vi "Read connections.vi"(8 "error in (no error)":errorcluster, 11 "Baseline Mocon piD-Tech plus in":refnum<class "Baseline Mocon piD-Tech plus.lvclass">) -> (0 "error out":errorcluster, 2 "Baseline-Mocon piD-TECH plus":T1, 3 "Baseline Mocon piD-Tech plus out":refnum<class "Baseline Mocon piD-Tech plus.lvclass">)   [LabVIEW 2011, in "Baseline Mocon piD-Tech plus.lvclass"]
uses:
  Baseline Mocon piD-Tech plus.lvclass
  Connections.ctl
  Baseline Mocon piD-Tech plus.lvclass/Baseline Mocon piD-Tech plus.ctl
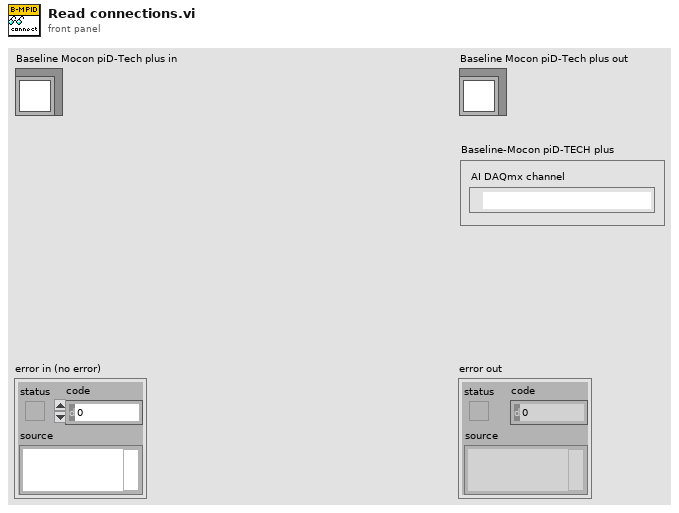
[diagram p1: front panel]
types:
  T1 = typedef "Baseline Mocon piD-Tech plus.lvclass/Connections.ctl" = cluster{"AI DAQmx channel":tag}
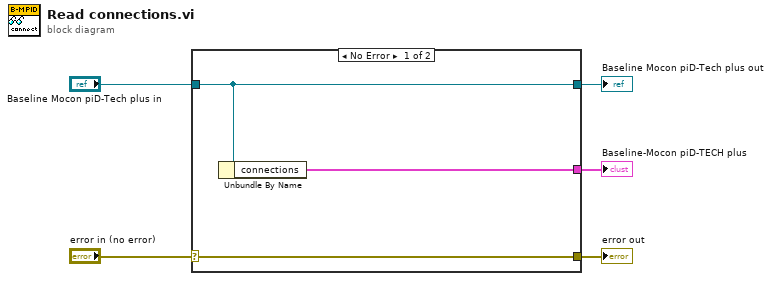
[diagram p0: block diagram]
diagram:
  n1 = case shown="No Error" "error in (no error)" {
    selector: "error in (no error)" -> [w8 w9]
    tunnel: [w8 w9] -> w4
    tunnel: [w7 w10] -> w2
    tunnel: "Baseline Mocon piD-Tech plus in" -> [w7 w10]
    tunnel: [w6 _] -> w1
    frame No Error {
      n2 = Unbundle By Name(w7) -> ("connections"=w6:T1)
    }
    frame Error {
    }
  }
  "error out" <- w4
  "Baseline Mocon piD-Tech plus out" <- w2
  "Baseline-Mocon piD-TECH plus" <- w1
